vi "Teleop.vi"(10 "Match Info":T1={"Autonomous Elapsed Seconds"=0.0, "TeleOp Elapsed Seconds"=0.0, "Disabled Elapsed Seconds"=0.0, "Visited Autonomous"=FALSE, "Visited TeleOp"=FALSE, "Visited Disabled"=FALSE, "Autonomous Settings"={"Autonomous Style"=enum."Independent", "VI Refnum"=refnum}}, 11 "Call Context":T2) -> ()   [LabVIEW 2012]
doc: "This VI is called for each TeleOp packet received from the DS where the robot is not disabled. It is often used to read from the joysticks and update I/O or to update setpoints for timed control loops. It should complete and return within 20 milliseconds or it may miss DS packets."
uses:
  <vilib>/Rock Robotics/WPI/DriverStation/WPI_DriverStationDerivedRobotMode.ctl
  <vilib>/Rock Robotics/WPI/DriverStation/WPI_DriverStationMatch Info.ctl
  Robot Global Data.vi
  <vilib>/Rock Robotics/WPI/Joystick/WPI_JoystickGetSetRefNum.vi
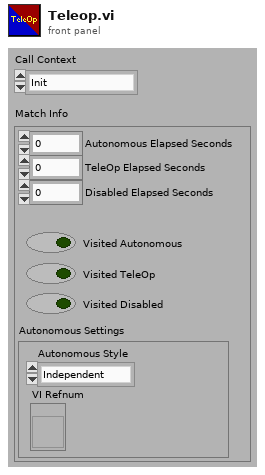
[diagram p1: front panel]
types:
  T1 = typedef "WPI_DriverStationMatch Info.ctl" = cluster{"Autonomous Elapsed Seconds":dbl, "TeleOp Elapsed Seconds":dbl, "Disabled Elapsed Seconds":dbl, "Visited Autonomous":bool, "Visited TeleOp":bool, "Visited Disabled":bool, "Autonomous Settings":cluster{"Autonomous Style":enum16{"Iterative", "Independent"}, "VI Refnum":refnum<vi>}}
  T2 = typedef "WPI_DriverStationDerivedRobotMode.ctl" = enum16{"Init", "Execute", "Stop"}
  T3 = typedef "WPI_JoystickDevRef.ctl" = cluster{"Device":T4}
  T4 = typedef "WPI_JoystickDeviceEnum.ctl" = enum16{"USB 1", "USB 2", "USB 3", "USB 4", "Kinect 1", "Kinect 2"}
  T5 = typedef "WPI_JoystickButtonState.ctl" = cluster{"Button 1":bool, "Button 2":bool, "Button 3":bool, "Button 4":bool, "Button 5":bool, "Button 6":bool, "Button 7":bool, "Button 8":bool, "Button 9":bool, "Button 10":bool, "Button 11":bool, "Button 12":bool}
  T6 = cluster{"axis 1 (x)":dbl, "axis 2 (y)":dbl, "axis 3 (throttle)":dbl, "axis 4":dbl, "axis 5":dbl, "axis 6":dbl}
  T7 = typedef "WPI_MotorControlDeviceRef.ctl" = cluster{"DeviceStatus":errorcluster, "Type":enum16{"PWM", "CAN"}, "PWM":cluster{"Digital Module":T8, "PWM Channel":T9, "DeadBand":T10}, "CAN":cluster{"Device Number":u8, "Control Mode":T11, "Semaphore":T12, "Max Vout":dbl}, "Invert":bool, "TransformRef":T13, "InvTransformRef":T13}
  T8 = typedef "FPGA_TypedefDigitalModule.ctl" = enum16{"Digital Module 1", "Digital Module 2"}
  T9 = typedef "FPGA_DIOPWMChannel.ctl" = enum8{"PWM 1", "PWM 2", "PWM 3", "PWM 4", "PWM 5", "PWM 6", "PWM 7", "PWM 8", "PWM 9", "PWM 10", "Invalid"}
  T10 = typedef "WPI_PWMDeadband.ctl" = cluster{"Name":string, "maxPositivePwm":i32, "minPositivePwm":i32, "centerPwm":i32, "maxNegativePwm":i32, "minNegativePwm":i32, "angularRange":u16}
  T11 = typedef "WPI_CANJaguar_ControlMode.ctl" = enum8{"Percent VBus", "Current", "Speed", "Position", "Voltage"}
  T12 = typedef "Semaphore RefNum" = refnum<k1>
  T13 = typedef "WPI_PWMTransform_ConPane.ctl" = refnum<vi>
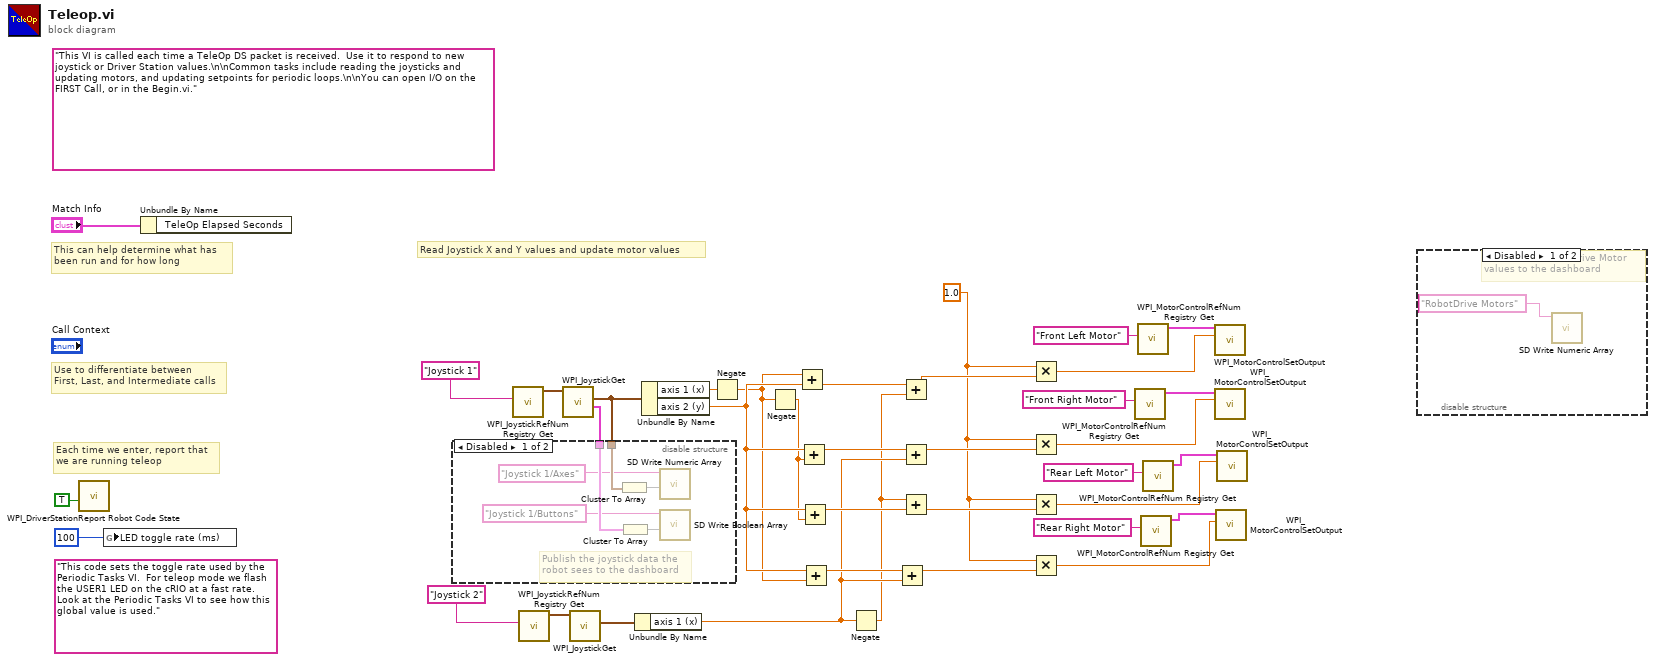
[diagram p0: block diagram]
diagram:
  w4 = 1.0
  (unwired) "This code sets the toggle rate used by the Periodic Tasks VI.  For teleop mode we flash the USER1 LED on the cRIO at a fast rate.  Look at the Periodic Tasks VI to see how this global value is used."
  (unwired) "This VI is called each time a TeleOp DS packet is received.  Use it to respond to new joystick or Driver Station values.\n\nCommon tasks include reading the joysticks and updating motors, and updating setpoints for periodic loops.\n\nYou can open I/O on the FIRST Call, or in the Begin.vi."
  # "Each time we enter, report that\nwe are running teleop"
  # "Use to differentiate between\nFirst, Last, and Intermediate calls"
  # "This can help determine what has\nbeen run and for how long"
  # "Read Joystick X and Y values and update motor values"
  n1 = call <vilib>:"WPI_DriverStationReport Robot Code State.vi"("TeleOp"=TRUE ("Autonomous")) -> ()  [unwired: 10 in, 1 out]
  n2 = global write "Robot Global Data.vi" "LED toggle rate (ms)"(u32 100 ("LED ms toggle rate")) -> ()
  n3 = Unbundle By Name("Match Info") -> ()  [unwired: 1 out]
  n4 = call <vilib>:"WPI_JoystickRefNum Registry Get.vi"("refnum name"="Joystick 1") -> ("JoystickDevRef"=w35:T3)  [unwired: 1 in, 9 out]
  n5 = call <vilib>:"WPI_JoystickRefNum Registry Get.vi"("refnum name"="Joystick 2") -> ("JoystickDevRef"=w29:T3)  [unwired: 1 in, 9 out]
  n6 = call <vilib>:"WPI_JoystickGet.vi"("JoystickDevRef"=w35) -> ("Buttons"=w32:T5, "Axes"=w31:T6)  [unwired: 1 in, 4 out]
  n7 = disable-structure shown="Disabled" {
    disable-tunnel: w32 -> [w43 _]
    disable-tunnel: w31 -> [w40 _]
    frame Disabled {
      # "Publish the joystick data the\nrobot sees to the dashboard"
      n8 = Cluster To Array(cluster=w40) -> (array=w39:dbl[])
      n9 = Cluster To Array(cluster=w43) -> (array=w42:bool[])
      n10 = call <vilib>:"SD Write Numeric Array.vi"("Numeric Array"=w39, "Name"="Joystick 1/Axes") -> ()  [unwired: 8 in, 2 out]
      n11 = call <vilib>:"SD Write Boolean Array.vi"("Boolean Array"=w42, "Name"="Joystick 1/Buttons") -> ()  [unwired: 8 in, 2 out]
    }
    frame Enabled {
    }
  }
  n12 = call <vilib>:"WPI_JoystickGet.vi"("JoystickDevRef"=w29) -> ("Axes"=w28:T6)  [unwired: 1 in, 5 out]
  n13 = Unbundle By Name(w28) -> ("axis 1 (x)"=w14:dbl)
  n14 = Unbundle By Name(w31) -> ("axis 1 (x)"=w3:dbl, "axis 2 (y)"=w23:dbl)
  n15 = Negate(x=w3) -> (-x=w1:dbl)
  n16 = Negate(x=w1) -> (-x=w2:dbl)
  n17 = Add(x=w1, y=w23) -> (x+y=w22:dbl)
  n18 = Add(x=w23, y=w2) -> (x+y=w21:dbl)
  n19 = Add(x=w23, y=w2) -> (x+y=w20:dbl)
  n20 = Add(x=w23, y=w1) -> (x+y=w19:dbl)
  n21 = Negate(x=w14) -> (-x=w13:dbl)
  n22 = Add(x=w19, y=w14) -> (x+y=w15:dbl)
  n23 = Add(x=w22, y=w13) -> (x+y=w18:dbl)
  n24 = Add(x=w21, y=w14) -> (x+y=w17:dbl)
  n25 = Add(x=w13, y=w20) -> (x+y=w16:dbl)
  n26 = Multiply(x=w4, y=w18) -> (x*y=w27:dbl)
  n27 = Multiply(x=w4, y=w17) -> (x*y=w26:dbl)
  n28 = Multiply(x=w4, y=w16) -> (x*y=w25:dbl)
  n29 = Multiply(x=w4, y=w15) -> (x*y=w24:dbl)
  n30 = call <vilib>:"WPI_MotorControlRefNum Registry Get.vi"("refnum name"="Front Right Motor") -> ("MotorControlDevRef"=w7:T7)  [unwired: 9 in, 1 out]
  n31 = call <vilib>:"WPI_MotorControlRefNum Registry Get.vi"("refnum name"="Front Left Motor") -> ("MotorControlDevRef"=w8:T7)  [unwired: 9 in, 1 out]
  n32 = call <vilib>:"WPI_MotorControlRefNum Registry Get.vi"("refnum name"="Rear Right Motor") -> ("MotorControlDevRef"=w5:T7)  [unwired: 9 in, 1 out]
  n33 = call <vilib>:"WPI_MotorControlRefNum Registry Get.vi"("refnum name"="Rear Left Motor") -> ("MotorControlDevRef"=w6:T7)  [unwired: 9 in, 1 out]
  n34 = call <vilib>:"WPI_MotorControlSetOutput.vi"("Output"=w27, "MotorControlDevRef"=w8) -> ()  [unwired: 7 in, 3 out]
  n35 = call <vilib>:"WPI_MotorControlSetOutput.vi"("Output"=w26, "MotorControlDevRef"=w7) -> ()  [unwired: 7 in, 3 out]
  n36 = call <vilib>:"WPI_MotorControlSetOutput.vi"("Output"=w24, "MotorControlDevRef"=w5) -> ()  [unwired: 7 in, 3 out]
  n37 = call <vilib>:"WPI_MotorControlSetOutput.vi"("Output"=w25, "MotorControlDevRef"=w6) -> ()  [unwired: 7 in, 3 out]
  n38 = disable-structure shown="Disabled" {
    frame Disabled {
      # "Publish the Robot Drive Motor\nvalues to the dashboard"
      n39 = call <vilib>:"SD Write Numeric Array.vi"("Name"="RobotDrive Motors") -> ()  [unwired: 9 in, 2 out]
    }
    frame Enabled {
    }
  }
